vi "Get Array of SBlocks.vi"(8 "error in (no error)":errorcluster, 11 "Sequence of SBlocks in":refnum<class "Sequence of SBlocks.lvclass">) -> (0 "error out":errorcluster, 3 "Sequence of SBlocks out":refnum<class "Sequence of SBlocks.lvclass">)   [LabVIEW 2020, in "TALOS.lvlib" / "Run Utilities.lvlib" / "Sequence of SBlocks.lvclass"]
uses:
  Sequence of SBlocks.lvclass
  Schedule Block/Schedule Block.lvclass
  Sequence of SBlocks.lvclass/Sequence of SBlocks.ctl
panel:
  out "Array of SBlocks":refnum<class "Schedule Block.lvclass">[](array[class])
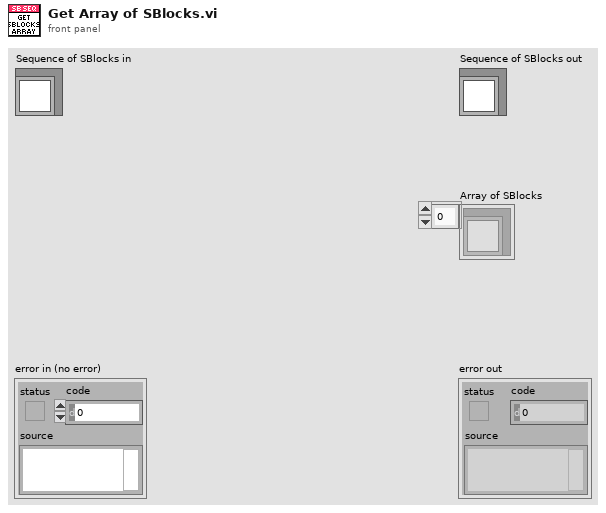
[diagram p1: front panel]
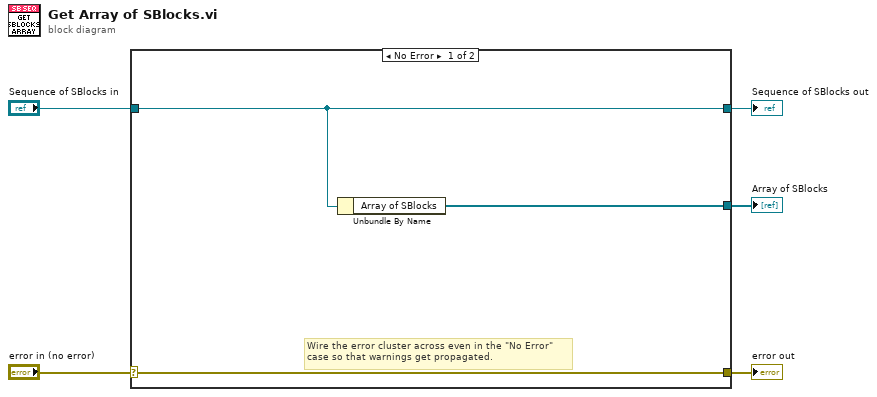
[diagram p0: block diagram]
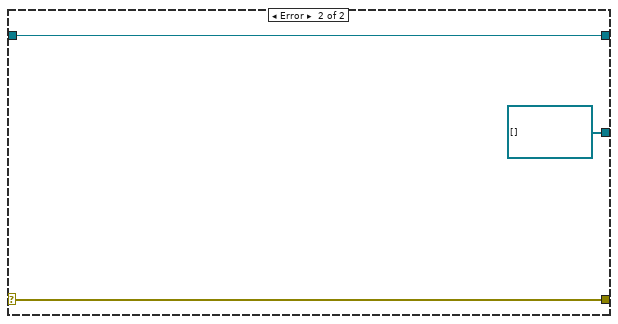
[diagram p2: hidden frame]
diagram:
  n1 = case shown="No Error" "error in (no error)" {
    selector: "error in (no error)" -> [w8 w11]
    tunnel: [w8 w11] -> w4
    tunnel: [w7 w10] -> w2
    tunnel: "Sequence of SBlocks in" -> [w7 w10]
    tunnel: [w6 refnum<class "Schedule Block.lvclass">[] [] ("Array of SBlocks")] -> w1
    frame No Error {
      # "Wire the error cluster across even in the \"No Error\"\ncase so that warnings get propagated."
      n2 = Unbundle By Name(w7) -> ("Array of SBlocks"=w6:refnum<class "Schedule Block.lvclass">[])
    }
    frame Error {
    }
  }
  "error out" <- w4
  "Sequence of SBlocks out" <- w2
  "Array of SBlocks" <- w1
